vi "Err check.vi"(8 "error in":errorcluster, 10 "Variant Control":variant, 11 "HW custom err":T1 items=["TX list"=10000, "TX length"=10001, "RX length"=10002]) -> (0 "error out":errorcluster)   [LabVIEW 2019, in "mmWave HW Control.lvlib"]
uses:
  mmWave HW Control.lvlib
  HW custom error.ctl
  <vilib>/Utility/error.llb/Error Cluster From Error Code.vi
  <vilib>/ErrorRing/Error Ring.xnode
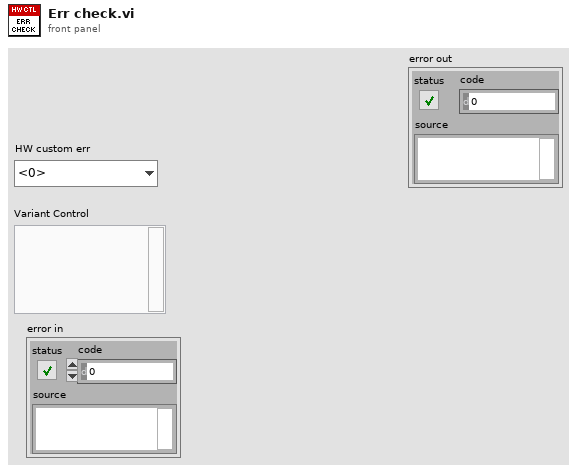
[diagram p1: front panel]
types:
  T1 = typedef "mmWave HW Control.lvlib/HW custom error.ctl" = u16
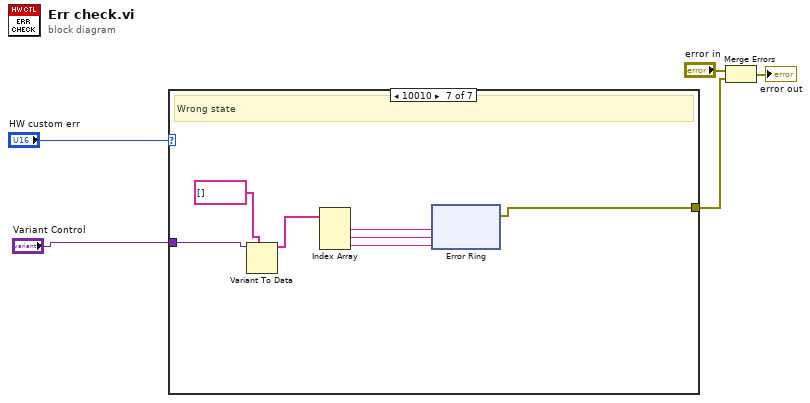
[diagram p0: block diagram]
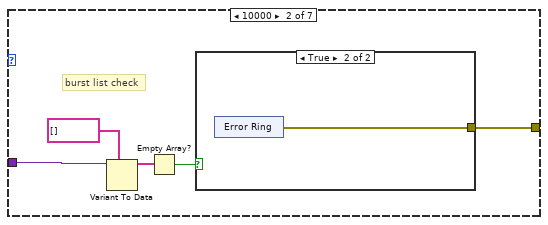
[diagram p3: hidden frame]
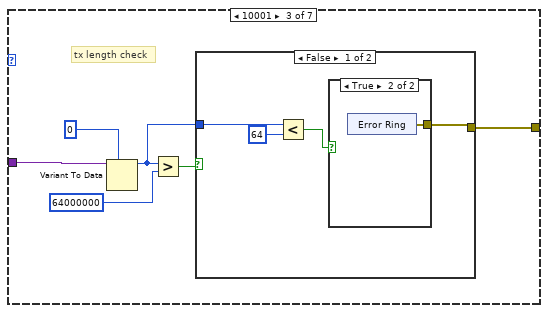
[diagram p5: hidden frame]
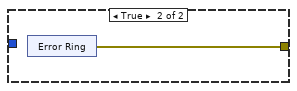
[diagram p7: hidden frame]
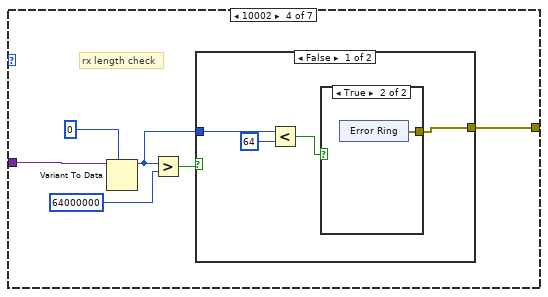
[diagram p8: hidden frame]
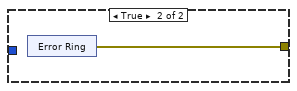
[diagram p10: hidden frame]
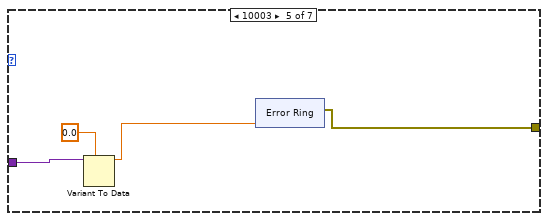
[diagram p11: hidden frame]
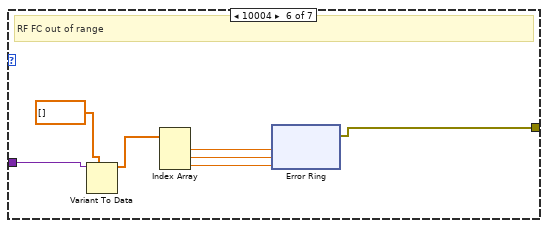
[diagram p12: hidden frame]
diagram:
  n1 = case shown="10010" "HW custom err" {
    tunnel: "Variant Control" -> [_ w10 w22 w44 w64 w78 w94]
    tunnel: [_ w6 w21 w43 w61 w72 w91] -> w3
    frame 0, Default {
    }
    frame 10000 {
      # "burst list check"
      n2 = Variant To Data(type=string[] [], Variant=w10) -> (data=w8:string[])  [unwired: 1 in, 1 out]
      n3 = Empty Array?(array=w8) -> (empty?=w7:bool)
      n4 = case shown="True" w7 {
        tunnel: [_ w11] -> w6
        frame False {
        }
        frame True {
          n5 = xnode "Error Ring"() -> ("error out"=w11:errorcluster)
        }
      }
    }
    frame 10001 {
      # "tx length check"
      n6 = Variant To Data(type=0, Variant=w22) -> (data=w17:i32)  [unwired: 1 in, 1 out]
      n7 = Greater?(x=w17, y=64000000) -> (0:w18:bool)
      n8 = case shown="False" w18 {
        tunnel: [w23 w33] -> w21
        tunnel: w17 -> [w26 _]
        frame False {
          n9 = Less?(x=w26, y=64) -> (x < y?=w24:bool)
          n10 = case shown="True" w24 {
            tunnel: [_ w27] -> w23
            frame False {
            }
            frame True {
              n11 = xnode "Error Ring"() -> ("error out"=w27:errorcluster)
            }
          }
        }
        frame True {
          n12 = xnode "Error Ring"() -> ("error out"=w33:errorcluster)
        }
      }
    }
    frame 10002 {
      # "rx length check"
      n13 = Variant To Data(type=0, Variant=w44) -> (data=w39:i32)  [unwired: 1 in, 1 out]
      n14 = Greater?(x=w39, y=64000000) -> (0:w40:bool)
      n15 = case shown="False" w40 {
        tunnel: [w45 w55] -> w43
        tunnel: w39 -> [w46 _]
        frame False {
          n16 = Less?(x=w46, y=64) -> (x < y?=w47:bool)
          n17 = case shown="True" w47 {
            tunnel: [_ w49] -> w45
            frame False {
            }
            frame True {
              n18 = xnode "Error Ring"() -> ("error out"=w49:errorcluster)
            }
          }
        }
        frame True {
          n19 = xnode "Error Ring"() -> ("error out"=w55:errorcluster)
        }
      }
    }
    frame 10003 {
      n20 = Variant To Data(type=0.0, Variant=w64) -> (data=w62:dbl)  [unwired: 1 in, 1 out]
      n21 = xnode "Error Ring"("parameter 0"=w62) -> ("error out"=w61:errorcluster)
    }
    frame 10004 {
      # "RF FC out of range"
      n22 = Variant To Data(type=dbl[] [], Variant=w78) -> (data=w76:dbl[])  [unwired: 1 in, 1 out]
      n23 = Index Array(array=w76) -> (element #1=w75:dbl, element #2=w74:dbl, element #3=w73:dbl)  [unwired: 3 in]
      n24 = xnode "Error Ring"("parameter 0"=w75, "parameter 1"=w74, "parameter 2"=w73) -> ("error out"=w72:errorcluster)
    }
    frame 10010 {
      # "Wrong state"
      n25 = Variant To Data(type=string[] [], Variant=w94) -> (data=w92:string[])  [unwired: 1 in, 1 out]
      n26 = Index Array(array=w92) -> (element #1=w90:string, element #2=w89:string, element #3=w88:string)  [unwired: 3 in]
      n27 = xnode "Error Ring"("parameter 0"=w90, "parameter 1"=w89, "parameter 2"=w88) -> ("error out"=w91:errorcluster)
    }
  }
  n28 = Merge Errors("error in", w3) -> (→"error out":errorcluster)
